vi "Read Attributes.vi"(11 "Set Single Device IED MicrogridID Msg":refnum<class "Set Single Device IED MicrogridID Msg.lvclass">) -> (2 "Payload":cluster{"IED_setMicrogridID":T1})   [LabVIEW 2018, in "Device Communication and Control Abstract Actor.lvlib" / "Set Single Device IED MicrogridID Msg.lvclass"]
uses:
  Set Single Device IED MicrogridID Msg.lvclass
  <vilib>/ORNL/CSEISMIC DDS/CSEISMIC DDS Base/Data Types/IED_setMicrogridID.ctl
  <vilib>/ORNL/CSEISMIC DDS/CSEISMIC DDS Base/Data Types/Controls/DeviceID.ctl
  Set Single Device IED MicrogridID Msg.lvclass/Set Single Device IED MicrogridID Msg.ctl
  <vilib>/ORNL/CSEISMIC DDS/CSEISMIC DDS Base/CSEISMIC DDS.lvclass
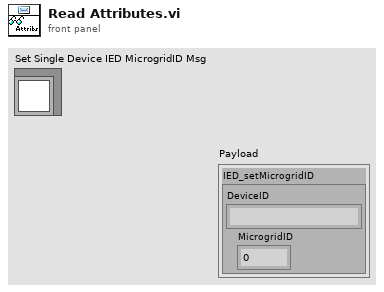
[diagram p1: front panel]
types:
  T1 = typedef "CSEISMIC DDS.lvlib/CSEISMIC DDS.lvclass/IED_setMicrogridID.ctl" = cluster{"DeviceID":T2, "MicrogridID":u8}
  T2 = typedef "CSEISMIC DDS.lvlib/CSEISMIC DDS.lvclass/DeviceID.ctl" = string
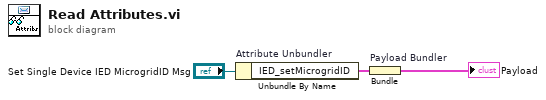
[diagram p0: block diagram]
diagram:
  n1 = Unbundle By Name "Attribute Unbundler"("Set Single Device IED MicrogridID Msg") -> ("IED_setMicrogridID"=w1:T1)
  n2 = Bundle "Payload Bundler"("IED_setMicrogridID"=w1) -> (→"Payload":cluster{"IED_setMicrogridID":T1})  [unwired: 1 in]
